vi "弯曲双线性分段.vi"(0 "数组－数值":dbl[](array[numeric]), 1 "数组－数值 2":dbl[](array[numeric])) -> (2 "子数组":dbl[](array[numeric]), 3 "子数组 2":dbl[](array[numeric]), 4 "子数组 3":dbl[](array[numeric]), 5 "子数组 4":dbl[](array[numeric]))   [LabVIEW 2016]
uses:
  <vilib>/Analysis/NI_AALPro.lvlib
panel:
  out "分界位置":i32
  out "斜率差":dbl[](array[numeric])
  out "斜率数据":dbl[](array[numeric])
  out "斜率":dbl
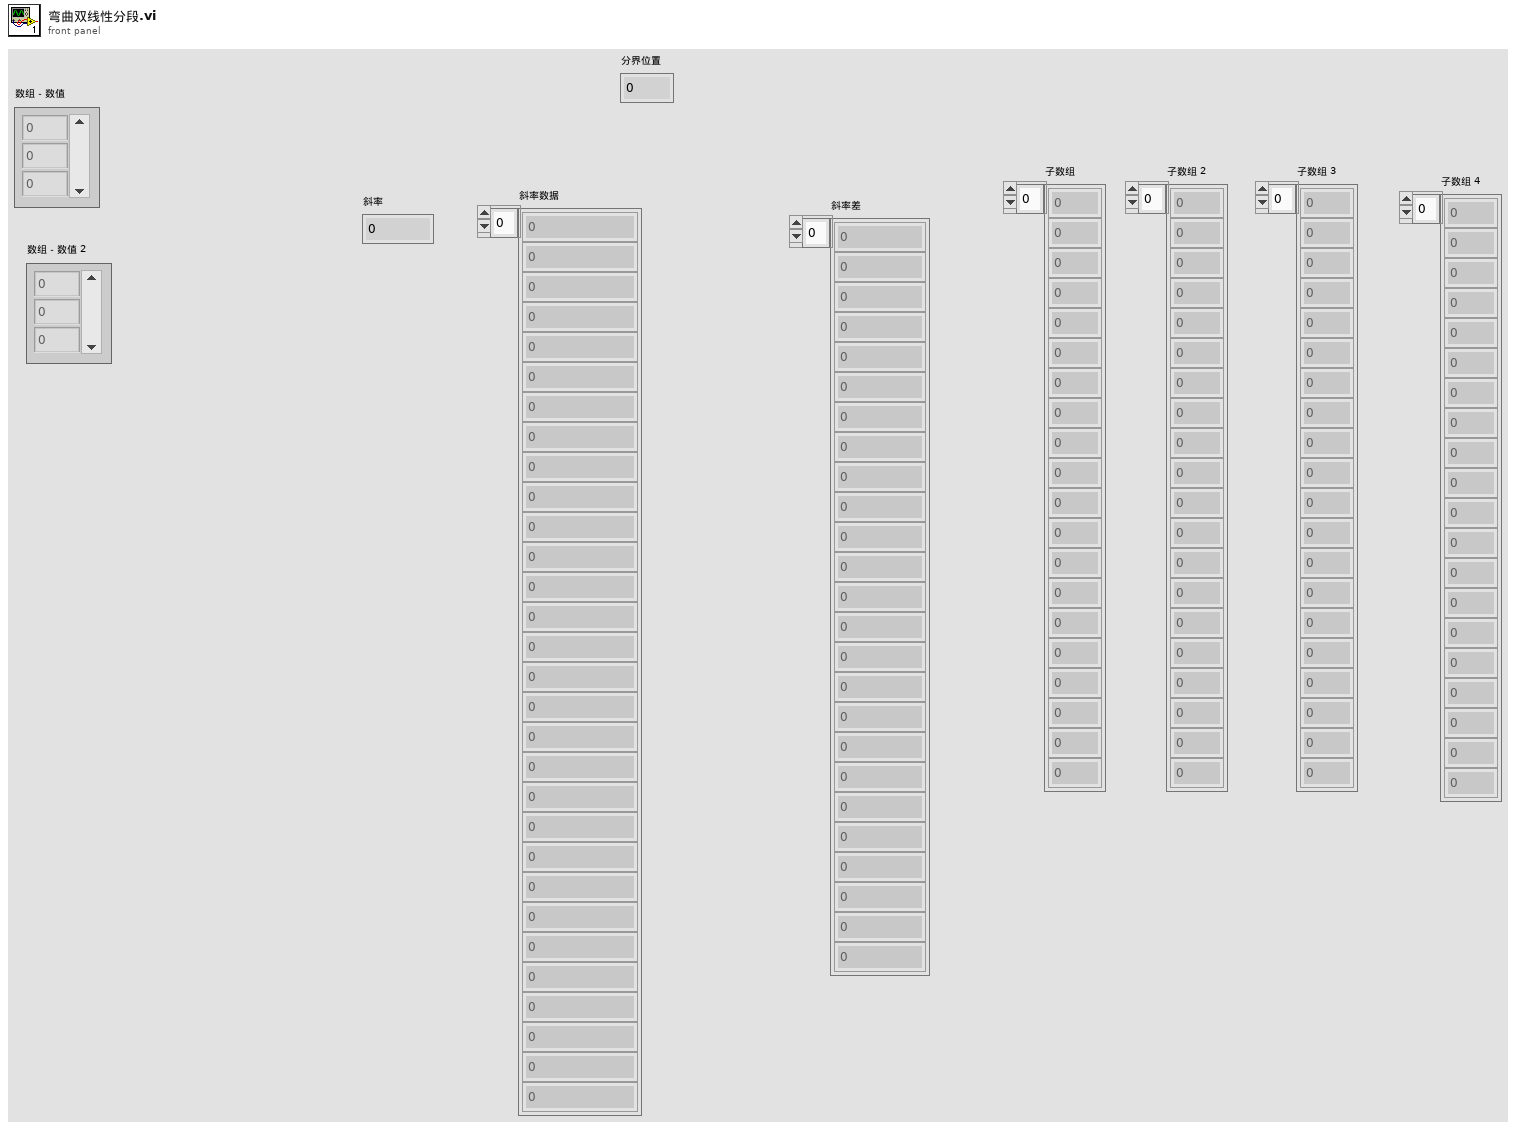
[diagram p1: front panel]
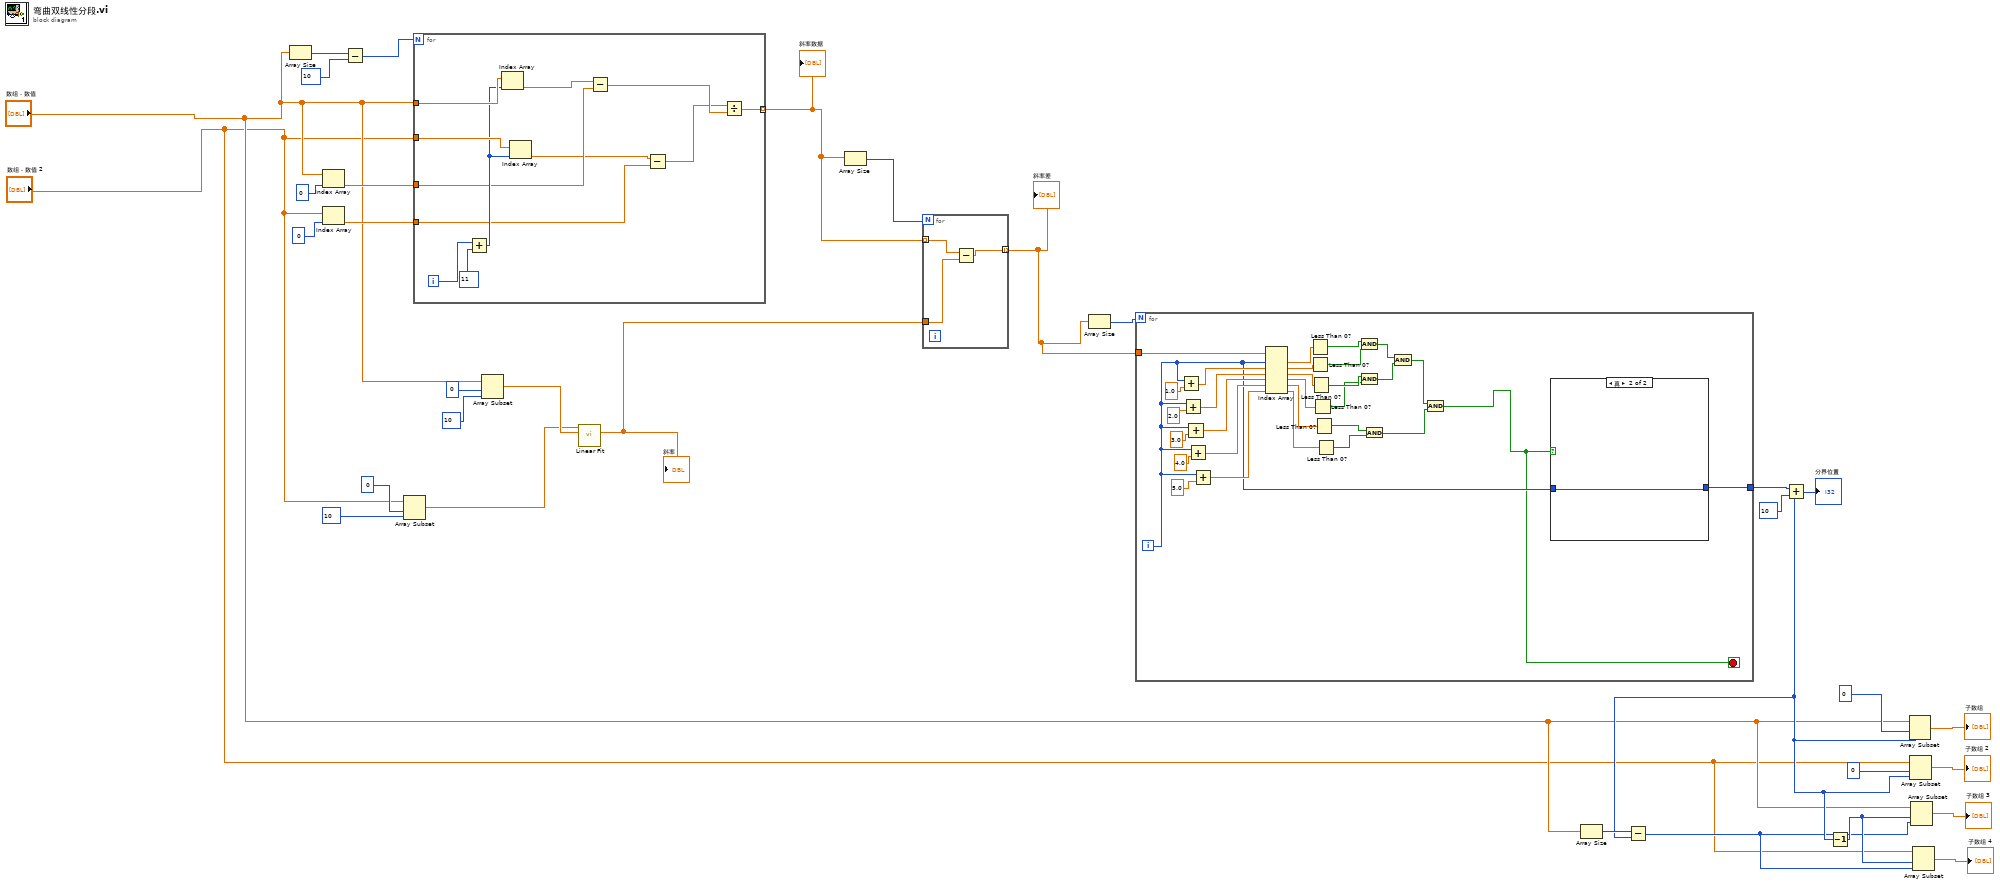
[diagram p0: block diagram]
diagram:
  n1 = Array Size(array="数组－数值") -> (size(s)=w32:i32)
  n2 = Index Array(array="数组－数值", index=0 ("索引")) -> (element=w27:dbl)
  n3 = Index Array(array="数组－数值 2", index=0 ("索引")) -> (element=w26:dbl)
  n4 = Subtract(x=w32, y=10) -> (x-y=w30:i32)
  n5 = Array Subset(array="数组－数值 2", index=0 ("索引"), length=10 ("长度")) -> (w15:dbl[])
  n6 = for {
    N: w30 -> [_]
    tunnel: "数组－数值" -> [w42]
    tunnel: "数组－数值 2" -> [w41]
    tunnel: w27 -> [w38]
    tunnel: w26 -> [w36]
    tunnel: [w35] -> w20 mode=indexing
    i -> [w44]
    n7 = Add(x=w44, y=11) -> (x+y=w40:i32)
    n8 = Index Array(array=w42, index=w40) -> (element=w39:dbl)
    n9 = Index Array(array=w41, index=w40) -> (element=w37:dbl)
    n10 = Subtract(x=w39, y=w38) -> (x-y=w34:dbl)
    n11 = Subtract(x=w37, y=w36) -> (x-y=w33:dbl)
    n12 = Divide(x=w33, y=w34) -> (x/y=w35:dbl)
  }
  "斜率数据" <- w20
  n13 = Array Subset(array="数组－数值", index=0 ("索引"), length=10 ("长度")) -> (w16:dbl[])
  n14 = call <vilib>:"Linear Fit.vi"("Y"=w15, "X"=w16) -> ("slope"=w19:dbl)  [unwired: 9 in, 4 out]
  "斜率" <- w19
  n15 = Array Size(array=w20) -> (size(s)=w21:i32)
  n16 = for {
    N: w21 -> [_]
    tunnel: w20 -> [w47] mode=indexing
    tunnel: w19 -> [w46]
    tunnel: [w45] -> w17 mode=indexing
    n17 = Subtract(x=w47, y=w46) -> (x-y=w45:dbl)
  }
  "斜率差" <- w17
  n18 = Array Size(array=w17) -> (size(s)=w18:i32)
  n19 = for {
    N: w18 -> [_]
    tunnel: w17 -> [w77]
    tunnel: [w65] -> w14
    i -> [w66]
    stop <- w48 stop-if-true
    n20 = Add(x=w66, y=1.0) -> (x+y=w71:dbl)
    n21 = Add(x=w66, y=2.0) -> (x+y=w70:dbl)
    n22 = Add(x=w66, y=3.0) -> (x+y=w69:dbl)
    n23 = Add(x=w66, y=4.0) -> (x+y=w68:dbl)
    n24 = Add(x=w66, y=5.0) -> (x+y=w67:dbl)
    n25 = Index Array(array=w77, index #1=w66, index #2=w71, index #3=w70, index #4=w69, index #5=w68, index #6=w67) -> (element #1=w64:dbl, element #2=w63:dbl, element #3=w62:dbl, element #4=w61:dbl, element #5=w60:dbl, element #6=w59:dbl)
    n26 = Less Than 0?(x=w64) -> (x < 0?=w58:bool)
    n27 = Less Than 0?(x=w63) -> (x < 0?=w57:bool)
    n28 = Less Than 0?(x=w62) -> (x < 0?=w56:bool)
    n29 = Less Than 0?(x=w61) -> (x < 0?=w55:bool)
    n30 = Less Than 0?(x=w60) -> (x < 0?=w54:bool)
    n31 = Less Than 0?(x=w59) -> (x < 0?=w53:bool)
    n32 = And(x=w58, y=w57) -> (x .and. y?=w52:bool)
    n33 = And(x=w56, y=w55) -> (x .and. y?=w51:bool)
    n34 = And(x=w54, y=w53) -> (x .and. y?=w50:bool)
    n35 = And(x=w52, y=w51) -> (x .and. y?=w49:bool)
    n36 = And(x=w49, y=w50) -> (x .and. y?=w48:bool)
    n37 = case shown="真" w48 {
      tunnel: w66 -> [_ w78]
      tunnel: [_ w78] -> w65
      frame False {
      }
      frame True {
      }
    }
  }
  n38 = Array Size(array="数组－数值") -> (size(s)=w9:i32)
  n39 = Add(x=w14, y=10) -> (x+y=w8:i32)
  "分界位置" <- w8
  n40 = Subtract(x=w9, y=w8) -> (x-y=w7:i32)
  n41 = Decrement(x=w8) -> (x-1=w10:i32)
  n42 = Array Subset(array="数组－数值", index=0 ("索引"), length=w8) -> (→"子数组":dbl[])
  n43 = Array Subset(array="数组－数值 2", index=0 ("索引"), length=w8) -> (→"子数组 2":dbl[])
  n44 = Array Subset(array="数组－数值", index=w10, length=w7) -> (→"子数组 3":dbl[])
  n45 = Array Subset(array="数组－数值 2", index=w10, length=w7) -> (→"子数组 4":dbl[])
